vi "Register Q and notifier.vi"(0 "Type":T1(ring), 1 "Action(GET)":enum16{"GET", "SET"}(ring), 7 "Name in":string, 9 "Data type":variant, 11 "error in (no error)":errorcluster) -> (4 "Numb Names":i32, 8 "Names":string[](array[string]), 10 "Types":variant[](array[variant]), 15 "error out":errorcluster)   [LabVIEW 2010]
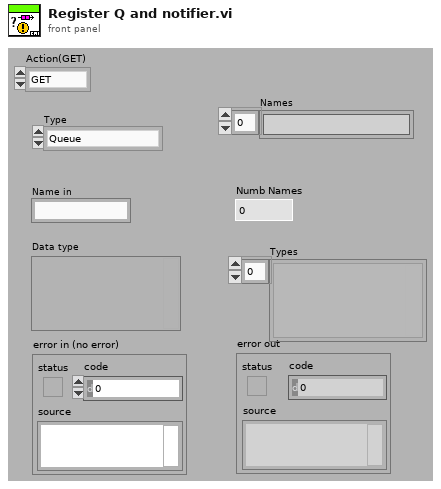
[diagram p1: front panel]
types:
  T1 = enum16{"Queue", "Notifier", "Semaphore", "Rendezvous"}
  T2 = cluster{"Queue":string[], "Notifier":string[], "Semaphore":string[], "Rendezvous":string[]}
  T3 = cluster{"Queue":variant[], "Notifier":variant[], "Semaphore":variant[], "Rendezvous":variant[]}
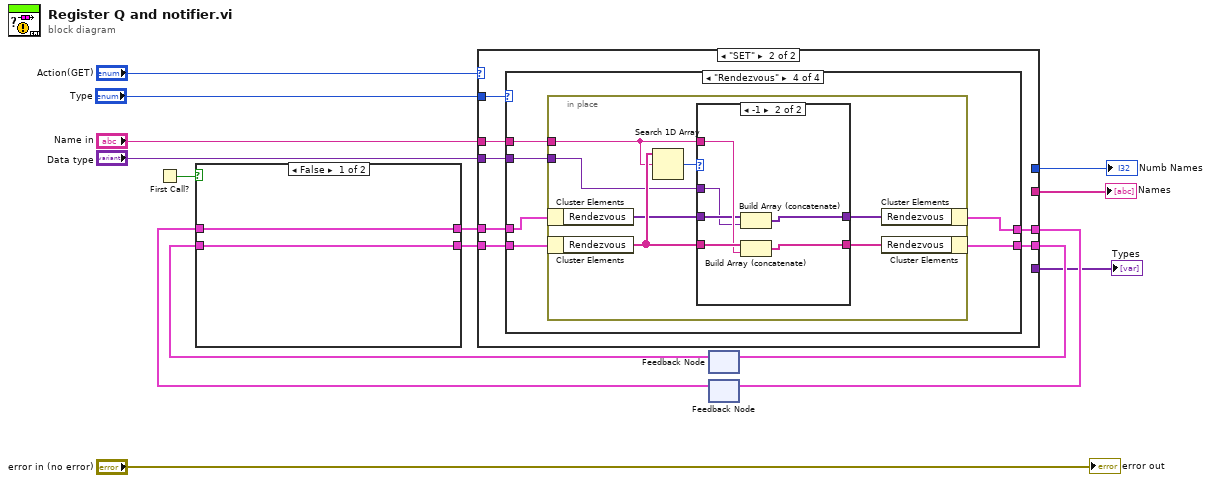
[diagram p0: block diagram]
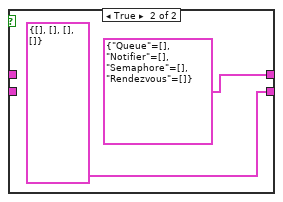
[diagram p2: hidden frame]
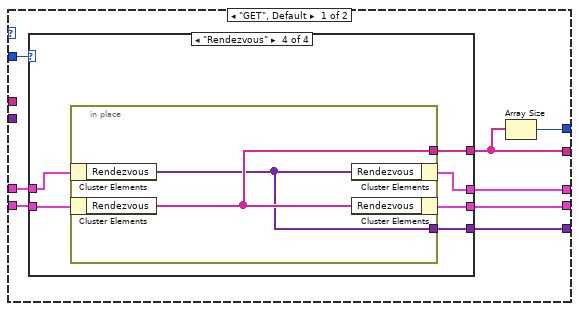
[diagram p3: hidden frame]
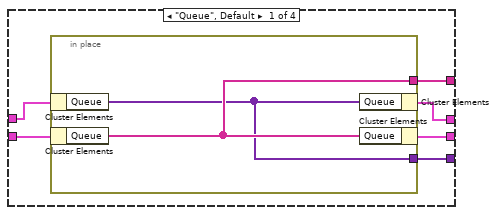
[diagram p4: hidden frame]
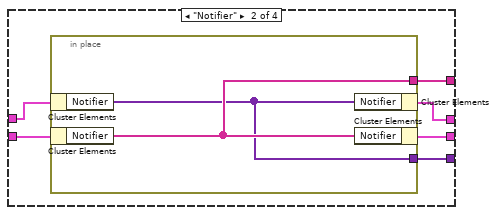
[diagram p5: hidden frame]
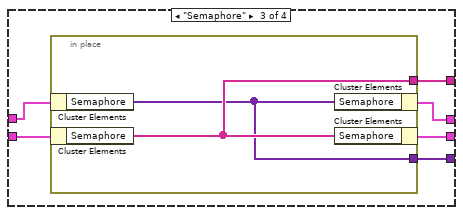
[diagram p6: hidden frame]
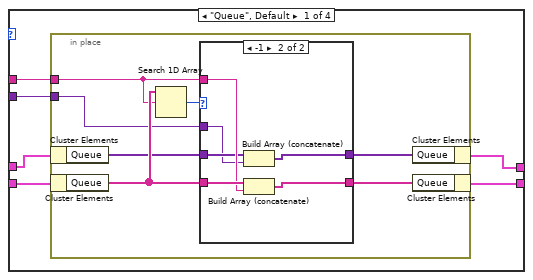
[diagram p7: hidden frame]
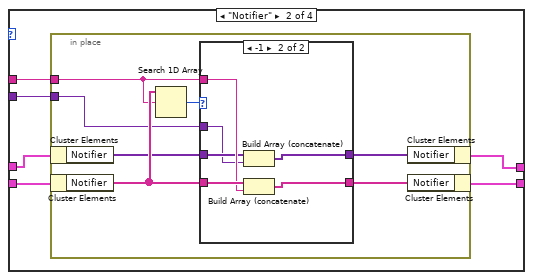
[diagram p9: hidden frame]
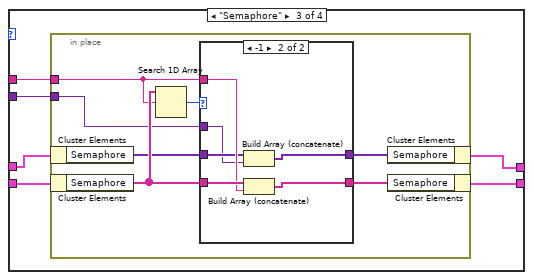
[diagram p11: hidden frame]
diagram:
  n1 = First Call?() -> (First Call?: T/F=w12:bool)
  n2 = feedback #1() -> (w13:T2)  [unwired: 1 in]
  n3 = feedback #2() -> (w2:T3)  [unwired: 1 in]
  n4 = case shown="False" w12 {
    tunnel: w13 -> [w17 _]
    tunnel: [w17 T2 {"Queue"=[], "Notifier"=[], "Semaphore"=[], "Rendezvous"=[]} ("output cluster")] -> w10
    tunnel: [w16 T3 {"Queue"=[], "Notifier"=[], "Semaphore"=[], "Rendezvous"=[]} ("output cluster")] -> w4
    tunnel: w2 -> [w16 _]
    frame False {
    }
    frame True {
    }
  }
  n5 = case shown="\"SET\"" "Action(GET)" {
    tunnel: [w26 w63] -> w11
    tunnel: w10 -> [w27 w65]
    tunnel: "Name in" -> [_ w64]
    tunnel: "Type" -> [w23 w66]
    tunnel: [w25 _] -> w7
    tunnel: [w24 _] -> w6
    tunnel: "Data type" -> [_ w62]
    tunnel: w4 -> [w22 w61]
    tunnel: [w21 w60] -> w3
    tunnel: [w20 _] -> w1
    frame "GET", Default {
      n6 = case shown="\"Rendezvous\"" w23 {
        tunnel: w27 -> [w32 w40 w48 w56]
        tunnel: [w33 w41 w49 w57] -> w26
        tunnel: [w31 w39 w47 w55] -> w25
        tunnel: w22 -> [w30 w38 w46 w54]
        tunnel: [w29 w37 w45 w53] -> w21
        tunnel: [w28 w36 w44 w52] -> w20
        frame "Queue", Default {
          n7 = in-place {
            in-place-border: [w35] -> w31
            in-place-border: [w34] -> w28
            n8 = in-place-cluster #3(w30) -> ("Queue"=w34:variant[])
            n9 = in-place-cluster #4(w32) -> ("Queue"=w35:string[])
            n10 = in-place-cluster #3("Queue"=w34) -> (w29:T3)
            n11 = in-place-cluster #4("Queue"=w35) -> (w33:T2)
          }
        }
        frame "Notifier" {
          n12 = in-place {
            in-place-border: [w43] -> w39
            in-place-border: [w42] -> w36
            n13 = in-place-cluster #5(w38) -> ("Notifier"=w42:variant[])
            n14 = in-place-cluster #6(w40) -> ("Notifier"=w43:string[])
            n15 = in-place-cluster #5("Notifier"=w42) -> (w37:T3)
            n16 = in-place-cluster #6("Notifier"=w43) -> (w41:T2)
          }
        }
        frame "Semaphore" {
          n17 = in-place {
            in-place-border: [w51] -> w47
            in-place-border: [w50] -> w44
            n18 = in-place-cluster #7(w46) -> ("Semaphore"=w50:variant[])
            n19 = in-place-cluster #8(w48) -> ("Semaphore"=w51:string[])
            n20 = in-place-cluster #7("Semaphore"=w50) -> (w45:T3)
            n21 = in-place-cluster #8("Semaphore"=w51) -> (w49:T2)
          }
        }
        frame "Rendezvous" {
          n22 = in-place {
            in-place-border: [w59] -> w55
            in-place-border: [w58] -> w52
            n23 = in-place-cluster #9(w54) -> ("Rendezvous"=w58:variant[])
            n24 = in-place-cluster #10(w56) -> ("Rendezvous"=w59:string[])
            n25 = in-place-cluster #9("Rendezvous"=w58) -> (w53:T3)
            n26 = in-place-cluster #10("Rendezvous"=w59) -> (w57:T2)
          }
        }
      }
      n27 = Array Size(array=w25) -> (size(s)=w24:i32)
    }
    frame "SET" {
      n28 = case shown="\"Rendezvous\"" w66 {
        tunnel: w65 -> [w70 w91 w112 w133]
        tunnel: w64 -> [w72 w93 w114 w135]
        tunnel: [w71 w92 w113 w134] -> w63
        tunnel: w62 -> [w67 w88 w109 w130]
        tunnel: w61 -> [w69 w90 w111 w132]
        tunnel: [w68 w89 w110 w131] -> w60
        frame "Queue", Default {
          n29 = in-place {
            in-place-border: w72 -> [w77]
            in-place-border: w67 -> [w73]
            n30 = in-place-cluster #11(w69) -> ("Queue"=w75:variant[])
            n31 = in-place-cluster #12(w70) -> ("Queue"=w78:string[])
            n32 = Search 1D Array(1D array=w78, element=w77) -> (index of element=w76:i32)  [unwired: 1 in]
            n33 = case shown="-1" w76 {
              tunnel: [w81 w87] -> w79
              tunnel: w78 -> [w81 w86]
              tunnel: w77 -> [_ w85]
              tunnel: w75 -> [w80 w84]
              tunnel: [w80 w83] -> w74
              tunnel: w73 -> [_ w82]
              frame 0, Default {
              }
              frame -1 {
                n34 = Build Array (concatenate)(w84, w82) -> (w83:variant[])
                n35 = Build Array (concatenate)(w86, w85) -> (w87:string[])
              }
            }
            n36 = in-place-cluster #11("Queue"=w74) -> (w68:T3)
            n37 = in-place-cluster #12("Queue"=w79) -> (w71:T2)
          }
        }
        frame "Notifier" {
          n38 = in-place {
            in-place-border: w93 -> [w98]
            in-place-border: w88 -> [w94]
            n39 = in-place-cluster #13(w90) -> ("Notifier"=w96:variant[])
            n40 = in-place-cluster #14(w91) -> ("Notifier"=w99:string[])
            n41 = Search 1D Array(1D array=w99, element=w98) -> (index of element=w97:i32)  [unwired: 1 in]
            n42 = case shown="-1" w97 {
              tunnel: [w102 w108] -> w100
              tunnel: w99 -> [w102 w107]
              tunnel: w98 -> [_ w106]
              tunnel: w96 -> [w101 w105]
              tunnel: [w101 w104] -> w95
              tunnel: w94 -> [_ w103]
              frame 0, Default {
              }
              frame -1 {
                n43 = Build Array (concatenate)(w105, w103) -> (w104:variant[])
                n44 = Build Array (concatenate)(w107, w106) -> (w108:string[])
              }
            }
            n45 = in-place-cluster #13("Notifier"=w95) -> (w89:T3)
            n46 = in-place-cluster #14("Notifier"=w100) -> (w92:T2)
          }
        }
        frame "Semaphore" {
          n47 = in-place {
            in-place-border: w114 -> [w119]
            in-place-border: w109 -> [w115]
            n48 = in-place-cluster #15(w111) -> ("Semaphore"=w117:variant[])
            n49 = in-place-cluster #16(w112) -> ("Semaphore"=w120:string[])
            n50 = Search 1D Array(1D array=w120, element=w119) -> (index of element=w118:i32)  [unwired: 1 in]
            n51 = case shown="-1" w118 {
              tunnel: [w123 w129] -> w121
              tunnel: w120 -> [w123 w128]
              tunnel: w119 -> [_ w127]
              tunnel: w117 -> [w122 w126]
              tunnel: [w122 w125] -> w116
              tunnel: w115 -> [_ w124]
              frame 0, Default {
              }
              frame -1 {
                n52 = Build Array (concatenate)(w126, w124) -> (w125:variant[])
                n53 = Build Array (concatenate)(w128, w127) -> (w129:string[])
              }
            }
            n54 = in-place-cluster #15("Semaphore"=w116) -> (w110:T3)
            n55 = in-place-cluster #16("Semaphore"=w121) -> (w113:T2)
          }
        }
        frame "Rendezvous" {
          n56 = in-place {
            in-place-border: w135 -> [w140]
            in-place-border: w130 -> [w136]
            n57 = in-place-cluster #17(w132) -> ("Rendezvous"=w138:variant[])
            n58 = in-place-cluster #18(w133) -> ("Rendezvous"=w141:string[])
            n59 = Search 1D Array(1D array=w141, element=w140) -> (index of element=w139:i32)  [unwired: 1 in]
            n60 = case shown="-1" w139 {
              tunnel: [w144 w150] -> w142
              tunnel: w141 -> [w144 w149]
              tunnel: w140 -> [_ w148]
              tunnel: w138 -> [w143 w147]
              tunnel: [w143 w146] -> w137
              tunnel: w136 -> [_ w145]
              frame 0, Default {
              }
              frame -1 {
                n61 = Build Array (concatenate)(w147, w145) -> (w146:variant[])
                n62 = Build Array (concatenate)(w149, w148) -> (w150:string[])
              }
            }
            n63 = in-place-cluster #17("Rendezvous"=w137) -> (w131:T3)
            n64 = in-place-cluster #18("Rendezvous"=w142) -> (w134:T2)
          }
        }
      }
    }
  }
  "Names" <- w7
  "Numb Names" <- w6
  "Types" <- w1
  n65 = feedback-in #1(w11) -> ()
  n66 = feedback-in #2(w3) -> ()
  "error out" <- "error in (no error)"
